vi "Slerp_interpolation.vi"(3 "quaternion 2":T1, 4 "ratio":dbl, 5 "quaternion 1":T1) -> (1 "interpolated quaternion":T1)   [LabVIEW 2024]
uses:
  <vilib>/Analysis/NI_AALBase.lvlib
  <vilib>/Analysis/baseanly.llb/Real Dot Product.vi
  <vilib>/robotics/Kinematics/Quaternion.ctl
  <vilib>/robotics/Kinematics/NI_Kinematics.lvlib
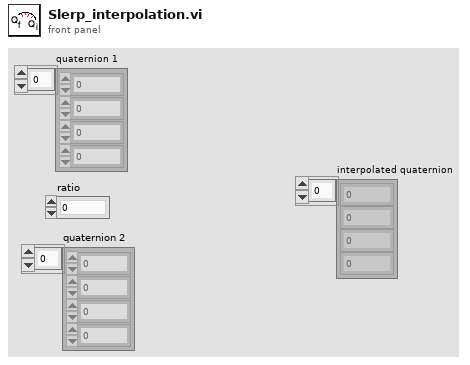
[diagram p1: front panel]
types:
  T1 = typedef "NI_Kinematics.lvlib/Quaternion.ctl" = dbl[]
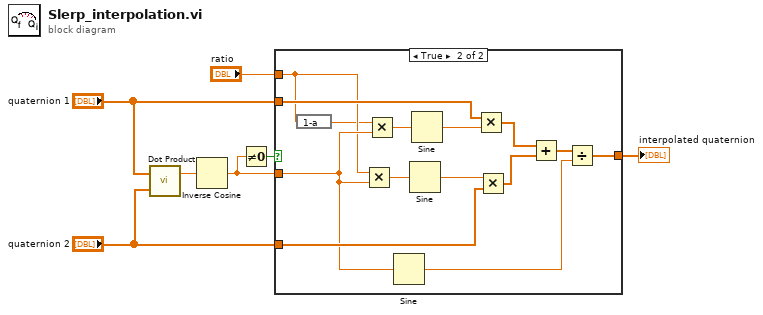
[diagram p0: block diagram]
diagram:
  n1 = call-poly <vilib>:"Dot Product.vi"("Y Vector"="quaternion 2", "X Vector"="quaternion 1") -> ("X * Y"=w7:dbl)  [unwired: 1 out]
  n2 = Inverse Cosine(1:w7) -> (0:w3:dbl)
  n3 = Not Equal To 0?(x=w3) -> (x != 0?=w4:bool)
  n4 = case shown="True" w4 {
    tunnel: "quaternion 1" -> [w8 w22]
    tunnel: "quaternion 2" -> [_ w21]
    tunnel: w3 -> [_ w12]
    tunnel: [w8 w13] -> w5
    tunnel: "ratio" -> [_ w10]
    frame False {
      # "q1 = q2"
    }
    frame True {
      n5 = expression code="1-a"(w10) -> (w9:dbl)
      n6 = Multiply(x=w10, y=w12) -> (x*y=w17:dbl)
      n7 = Multiply(x=w9, y=w12) -> (x*y=w20:dbl)
      n8 = Sine(x=w12) -> (sin(x)=w11:dbl)
      n9 = Sine(x=w17) -> (sin(x)=w18:dbl)
      n10 = Sine(x=w20) -> (sin(x)=w19:dbl)
      n11 = Multiply(x=w22, y=w19) -> (x*y=w16:T1)
      n12 = Multiply(x=w18, y=w21) -> (x*y=w15:T1)
      n13 = Add(x=w16, y=w15) -> (x+y=w14:T1)
      n14 = Divide(x=w14, y=w11) -> (x/y=w13:T1)
    }
  }
  "interpolated quaternion" <- w5
